vi "initialise.vi"(8 "error in (no error)":errorcluster, 11 "GenericPlugin in":refnum<class "StageDL090409Scaffold.lvclass">) -> (0 "error out":errorcluster, 3 "GenericPlugin out":refnum<class "StageDL090409Scaffold.lvclass">)   [LabVIEW 2010, in "StageDL090409Scaffold.lvclass"]
doc: "The dynamic dispatch-version of this VI initalises the plug-in object by allocating and initalising any dynamic resources need."
uses:
  StageDL090409Scaffold.lvclass
  GenericStage/GenericStage/GenericStage.lvclass
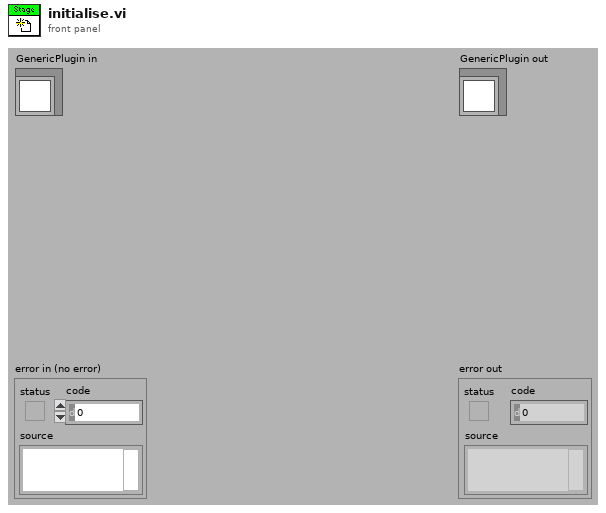
[diagram p1: front panel]
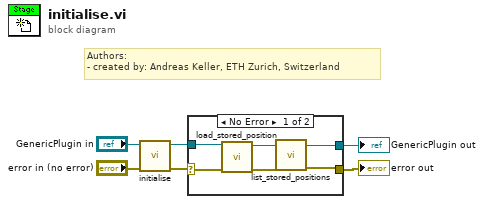
[diagram p0: block diagram]
diagram:
  # "Authors: \n- created by: Andreas Keller, ETH Zurich, Switzerland"
  n1 = call-parent "initialise.vi"("error in (no error)"="error in (no error)", "GenericPlugin in"="GenericPlugin in") -> ("error out"=w4:errorcluster, "GenericPlugin out"=w2:refnum<class "StageDL090409Scaffold.lvclass">)  [unwired: 8 in]
  n2 = case shown="No Error" w4 {
    selector: w4 -> [w12 w13]
    tunnel: [w9 w13] -> w3
    tunnel: w2 -> [w11 w14]
    tunnel: [w7 w14] -> w1
    frame No Error {
      n3 = call-dynamic "load_stored_position.vi"("error in (no error)"=w12, "StageDL090409Scaffold in"=w11) -> ("error out"=w10:errorcluster, "StageDL090409Scaffold out"=w8:refnum<class "StageDL090409Scaffold.lvclass">)  [unwired: 8 in]
      n4 = call-dynamic "list_stored_positions.vi"("error in (no error)"=w10, "StageDL090409Scaffold in"=w8) -> ("error out"=w9:errorcluster, "StageDL090409Scaffold out"=w7:refnum<class "StageDL090409Scaffold.lvclass">)  [unwired: 8 in]
    }
    frame Error {
    }
  }
  "error out" <- w3
  "GenericPlugin out" <- w1
